vi "getReferenceDomainId.vi"(8 "error in (no error)":errorcluster, 11 "IReferenceDomainInfo in":refnum<class "IReferenceDomainInfo.lvclass">) -> (0 "error out":errorcluster, 2 "DomainID out":string, 3 "IReferenceDomainInfo out":refnum<class "IReferenceDomainInfo.lvclass">)   [LabVIEW 2022 SP3, in "openDAQ.lvlib" / "IBaseObject.lvlib" / "IReferenceDomainInfo.lvlib" / "IReferenceDomainInfo.lvclass"]
uses:
  <instrlib>/openDAQ/Public/Classes/IReferenceDomainInfo/IReferenceDomainInfo.lvclass
  <instrlib>/openDAQ/Public/Classes/IReferenceDomainInfo/IReferenceDomainInfo.lvclass/IReferenceDomainInfo.ctl
  <instrlib>/openDAQ/Public/Classes/daqCoreTypes/IString/IString.lvclass
  <instrlib>/openDAQ/Binaries/Windows/x86/copendaq32.dll
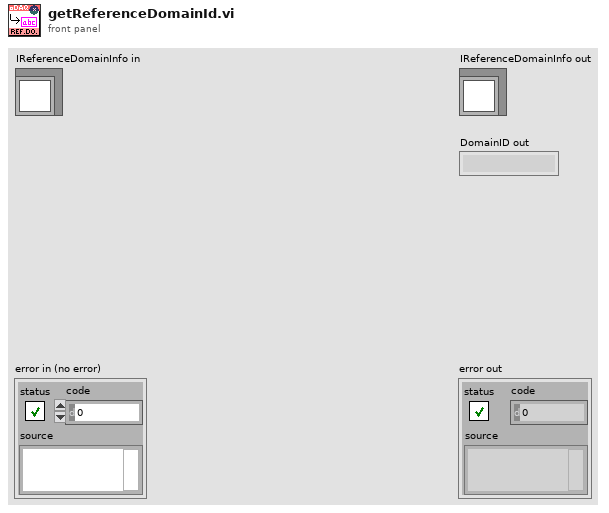
[diagram p1: front panel]
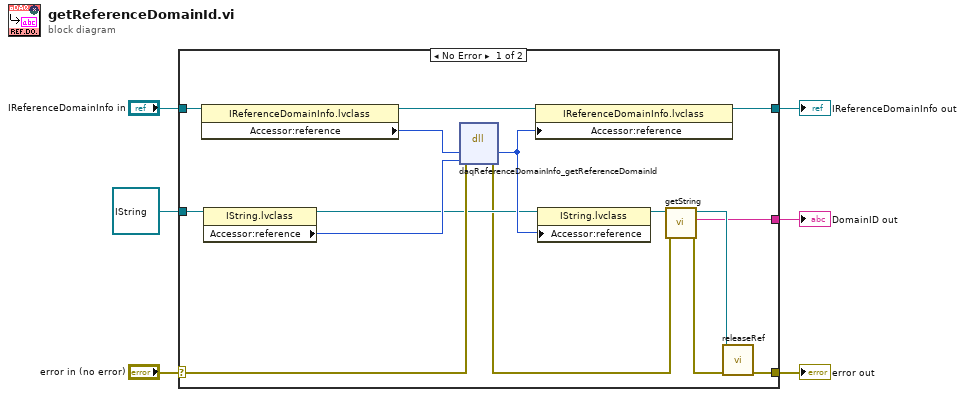
[diagram p0: block diagram]
diagram:
  n1 = case shown="No Error" "error in (no error)" {
    selector: "error in (no error)" -> [w17 w23]
    tunnel: [w9 w23] -> w5
    tunnel: [w15 w22] -> w3
    tunnel: "IReferenceDomainInfo in" -> [w18 w22]
    tunnel: refnum<class "IString.lvclass"> refnum ("openDAQ.lvlib:daqCoreTypes.lvlib:IString.lvclass") -> [w14 _]
    tunnel: [w7 _] -> w1
    frame No Error {
      n2 = property class="IReferenceDomainInfo.lvclass"(reference=w18) -> (reference out=w16:refnum<class "IReferenceDomainInfo.lvclass">, "Accessor:reference"=w21:i64)  [unwired: 1 in, 1 out]
      n3 = property class="IString.lvclass"(reference=w14) -> (reference out=w13:refnum<class "IString.lvclass">, "Accessor:reference"=w20:i64)  [unwired: 1 in, 1 out]
      n4 = dll-call lib="C:/Program Files (x86)/National Instruments/LabVIEW 2022/instr.lib/openDAQ/Binaries/Windows/x86/copendaq*.*" fn="daqReferenceDomainInfo_getReferenceDomainId"(error in=w17, "referenceDomainInfo"=w21, "domainID"=w20) -> (error out=w11:errorcluster, "referenceDomainInfo"=w19:i64)  [unwired: 4 in, 1 out]
      n5 = property class="IReferenceDomainInfo.lvclass"(reference=w16, "Accessor:reference"=w19) -> (reference out=w15:refnum<class "IReferenceDomainInfo.lvclass">)  [unwired: 1 in, 1 out]
      n6 = property class="IString.lvclass"(reference=w13, "Accessor:reference"=w19) -> (reference out=w12:refnum<class "IString.lvclass">)  [unwired: 1 in, 1 out]
      n7 = call <instrlib>:"getString.vi"("error in (no error)"=w11, "IString in"=w12) -> ("error out"=w10:errorcluster, "String out"=w7:string, "IString out"=w8:refnum<class "IString.lvclass">)  [unwired: 7 in]
      n8 = call-dynamic "releaseRef.vi"("error in (no error)"=w10, "IBaseObject in"=w8) -> ("error out"=w9:errorcluster)  [unwired: 9 in]
    }
    frame Error {
    }
  }
  "error out" <- w5
  "IReferenceDomainInfo out" <- w3
  "DomainID out" <- w1
